vi "Reset_All_Relay.vi"(8 "error in (no error)":errorcluster caption="entrée d'erreur (pas d'erreur)", 11 "Class Relay_Board 16_Relay_CH340 en entrée":refnum<class "Class Relay_Board 16_Relay_Acer_Micro.lvclass">) -> (0 "error out":errorcluster caption="sortie d'erreur", 3 "Class Relay_Board 16_Relay_CH340 en sortie":refnum<class "Class Relay_Board 16_Relay_Acer_Micro.lvclass">)   [LabVIEW 2020, in "Library Instrument & Equipement.lvlib" / "Library Relay_Board.lvlib" / "Class Relay_Board 16_Relay_Acer_Micro.lvclass"]
uses:
  Class Relay_Board 16_Relay_Acer_Micro.lvclass
  Class Relay_Board 16_Relay_Acer_Micro.lvclass/Class Relay_Board 16_Relay_Acer_Micro.ctl
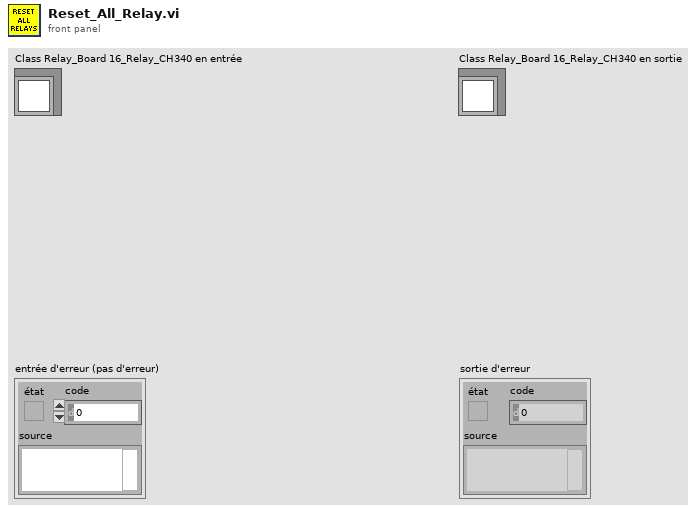
[diagram p1: front panel]
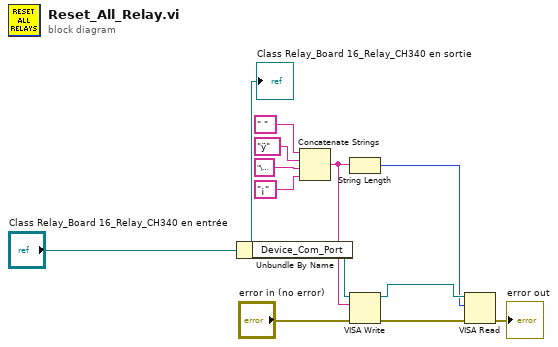
[diagram p0: block diagram]
diagram:
  n1 = Unbundle By Name("Class Relay_Board 16_Relay_CH340 en entrée") -> ("Device_Com_Port"=w11:refnum<visa-resource-name>)
  n2 = Concatenate Strings(" " ("chaîne"), "ÿ" ("chaîne"), "\u0000" ("chaîne"), "¡" ("chaîne")) -> (w4:string)
  n3 = String Length(string=w4) -> (length=w3:i32)
  n4 = VISA Write(VISA resource name=w11, write buffer=w4, error in (no error)="error in (no error)") -> (VISA resource name out=w5:refnum<visa-resource-name>, error out=w1:errorcluster)  [unwired: 1 out]
  n5 = VISA Read(VISA resource name=w5, byte count=w3, error in (no error)=w1) -> (error out=→"error out":errorcluster)  [unwired: 3 out]
  "Class Relay_Board 16_Relay_CH340 en sortie" <- "Class Relay_Board 16_Relay_CH340 en entrée"
